vi "Get Debug Flags.vi"(11 "Pool in":refnum<class "Pool.lvclass">) -> (2 "FIFO Debug Flags":refnum<class "Debug Flags FIFO.lvclass">, 3 "Pool out":refnum<class "Pool.lvclass">)   [LabVIEW 2017, in "Data Sharing Framework Engine.lvlib" / "Pool.lvclass"]
uses:
  Pool.lvclass
  Source/Data Sharing Framework Core/Engine/Debug/Debug Flags FIFO/Debug Flags FIFO.lvclass
  Pool.lvclass/Pool.ctl
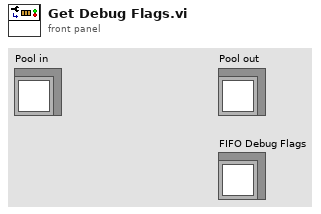
[diagram p1: front panel]
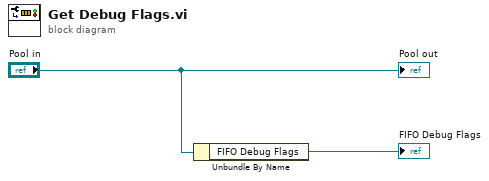
[diagram p0: block diagram]
diagram:
  n1 = Unbundle By Name("Pool in") -> ("FIFO Debug Flags"=→"FIFO Debug Flags":refnum<class "Debug Flags FIFO.lvclass">)
  "Pool out" <- "Pool in"
